vi "State Build.vi"(8 "error in (no error)":errorcluster, 9 "Parameters":variant, 11 "State":string) -> (0 "error out":errorcluster, 3 "State Out":T1)   [LabVIEW 2013, in "State Machine Lib.lvlib"]
doc: "Builds state cluster from state string and optional parameter (variant)"
uses:
  State Machine Lib.lvlib
  STATE cluster.ctl
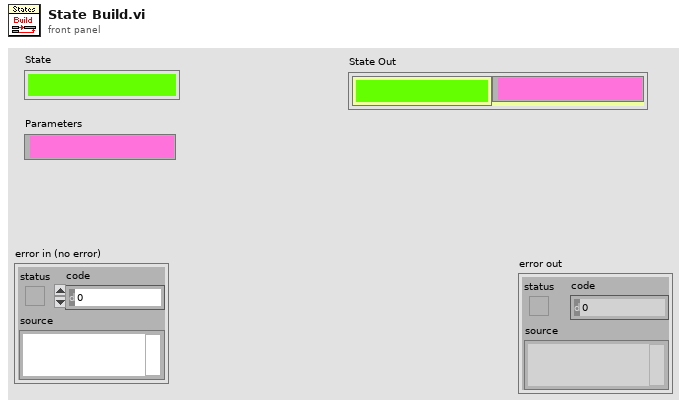
[diagram p1: front panel]
types:
  T1 = typedef "State Machine Lib.lvlib/STATE cluster.ctl" = cluster{"State":string, "Parameters":variant}
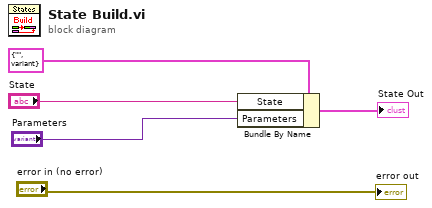
[diagram p0: block diagram]
diagram:
  n1 = Bundle By Name(cluster=T1 {"State"="", "Parameters"=variant} ("State Out"), "State"="State", "Parameters"="Parameters") -> (→"State Out":T1)
  "error out" <- "error in (no error)"
